vi "WD_Block_Move0515.vi"(7 "站點(記錄用)":string="790", 8 "error in (no error)":errorcluster, 9 "離開目標":i16, 10 "目前站點":i16, 11 "DBLink":string) -> (2 "workplace_data":cluster{"條碼R":string, "條碼L":string})   [LabVIEW 2019]
panel:
  # "此id為該位置檔快放行，把資料移至移動中"
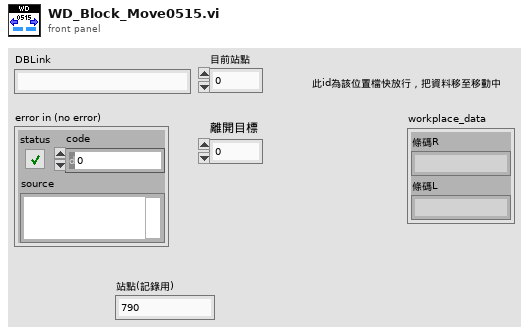
[diagram p1: front panel]
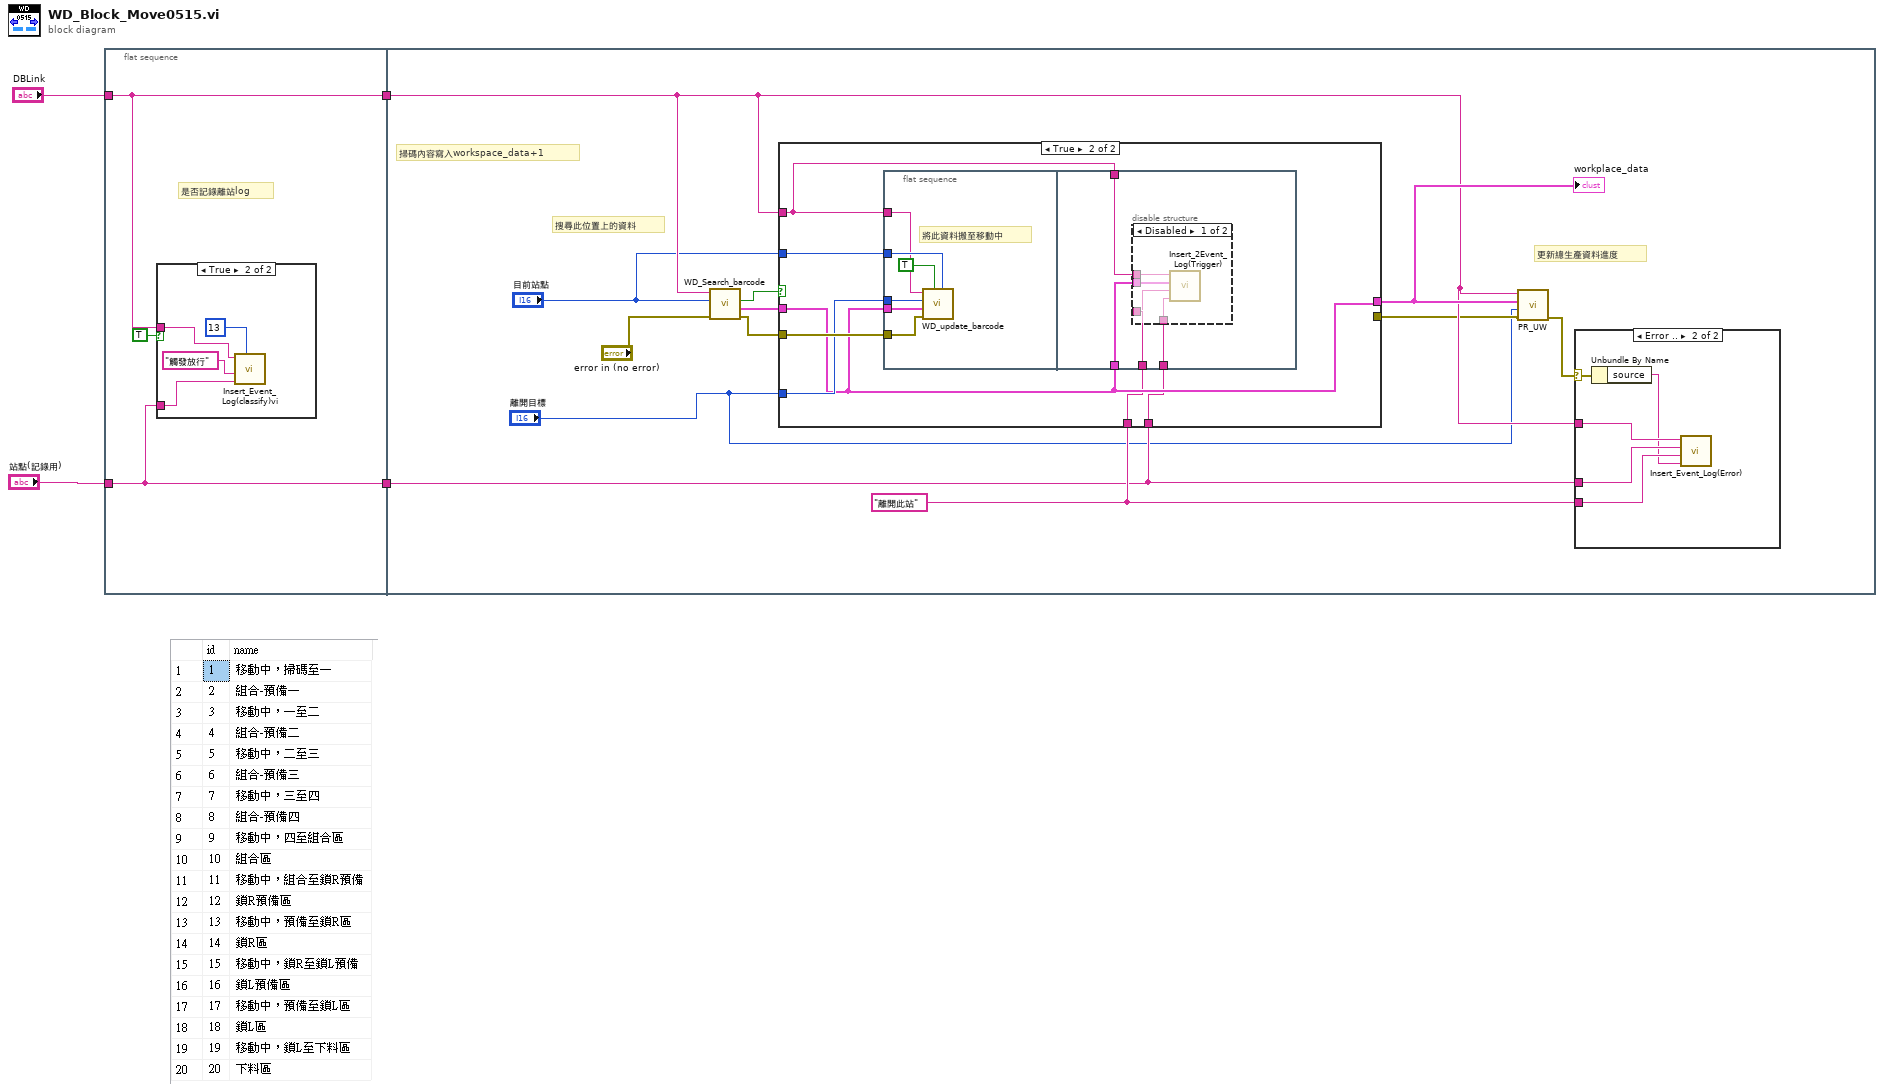
[diagram p0: block diagram]
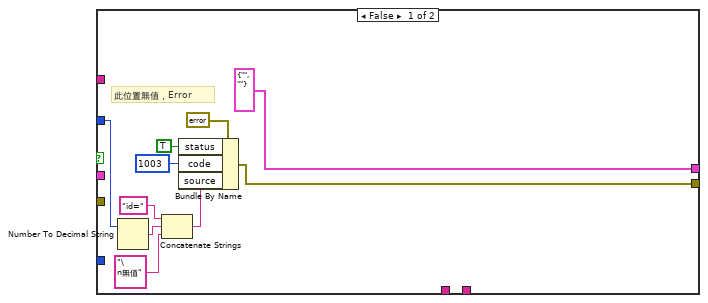
[diagram p4: hidden frame]
diagram:
  n1 = flat-sequence {
    tunnel: "站點(記錄用)" -> [w6]
    tunnel: "DBLink" -> [w7]
    tunnel: [w7] -> w2
    tunnel: [w6] -> w1
    tunnel: w2 -> [w17]
    tunnel: w1 -> [w15]
    frame #0 {
      # "是否記錄離站log"
      n2 = case shown="True" TRUE {
        tunnel: w7 -> [_ w9]
        tunnel: w6 -> [_ w8]
        frame False {
        }
        frame True {
          n3 = call "Insert_Event_Log(classify)vi.vi"("classify"=i16 13, "data"=w8, "message"="觸發放行", "DBlink"=w9) -> ()  [unwired: 7 in, 1 out]
        }
      }
    }
    frame #1 {
      w16 = "離開此站" ("message")
      # "搜尋此位置上的資料"
      # "更新總生產資料進度"
      # "掃碼內容寫入workspace_data+1"
      n4 = call "WD_Search_barcode.vi"("error in (no error)"="error in (no error)", "workplace_name_id"="目前站點", "DBlink"=w17) -> ("error out"=w23:errorcluster, "workplace_data"=w22:cluster{"條碼R":string, "條碼L":string}, "找到"=w21:bool)  [unwired: 5 in, 1 out]
      n5 = case shown="True" w21 {
        tunnel: w17 -> [_ w41]
        tunnel: w22 -> [_ w42]
        tunnel: w23 -> [_ w45]
        tunnel: "目前站點" -> [w35 w44]
        tunnel: "離開目標" -> [_ w43]
        tunnel: [cluster{"條碼A":string, "條碼B":string} {"條碼A"="", "條碼B"=""} ("workplace_data") w42] -> w19
        tunnel: w15 -> [_ w40]
        tunnel: w16 -> [_ w39]
        tunnel: [w29 _] -> w14
        frame False {
          # "此位置無值，Error"
          n6 = Number To Decimal String(number=w35) -> (decimal integer string=w33:string)  [unwired: 1 in]
          n7 = Concatenate Strings("id=", w33, "\n無值" ("string")) -> (w31:string)
          n8 = Bundle By Name(cluster=errorcluster {"status"=FALSE, "code"=0, "source"=""} ("error out"), "status"=TRUE, "code"=1003, "source"=w31) -> (w29:errorcluster)
        }
        frame True {
          n9 = flat-sequence {
            tunnel: w45 -> [w51]
            tunnel: w44 -> [w49]
            tunnel: w43 -> [w48]
            tunnel: w41 -> [w47]
            tunnel: w42 -> [w46]
            tunnel: w42 -> [w55]
            tunnel: w41 -> [w54]
            tunnel: w40 -> [w53]
            tunnel: w39 -> [w52]
            frame #0 {
              # "將此資料搬至移動中"
              n10 = call "WD_update_barcode.vi"("NULL: workplace_id"=w49, "Set null"=TRUE, "error in (no error)"=w51, "Workplace data"=w46, "workplace_id"=w48, "DBlink"=w47) -> ()  [unwired: 6 in]
            }
            frame #1 {
              n11 = disable-structure shown="Disabled" {
                disable-tunnel: w55 -> [w59 _]
                disable-tunnel: w54 -> [w58 _]
                disable-tunnel: w53 -> [w57 _]
                disable-tunnel: w52 -> [w56 _]
                frame Disabled {
                  n12 = call "Insert_2Event_Log(Trigger).vi"("data"=w57, "message"=w56, "output cluster"=w59, "DBlink"=w58) -> ()  [unwired: 8 in]
                }
                frame Enabled {
                }
              }
            }
          }
        }
      }
      "workplace_data" <- w19
      n13 = call "PR_UW .vi"("error in (no error)"=w14, "[workplace_id]"="離開目標", "當前工位資料"=w19, "DBlink"=w17) -> ("error out"=w18:errorcluster)  [unwired: 7 in]
      n14 = case shown="Error .." w18 {
        selector: w18 -> [_ w25]
        tunnel: w17 -> [_ w28]
        tunnel: w15 -> [_ w27]
        tunnel: w16 -> [_ w26]
        frame No Error {
        }
        frame Error {
          n15 = Unbundle By Name(w25) -> ("source"=w24:string)
          n16 = call "Insert_Event_Log(Error).vi"("data"=w24, "message"=w26, "id"=w27, "DBlink"=w28) -> ()  [unwired: 8 in]
        }
      }
    }
  }
